vi "BigArraySandbox.vi"() -> ()   [LabVIEW 2016]
panel:
  in  "other Y axis":enum16{"A", "B", "C", "D"}(ring)=enum."D"
  in  "Z Ring":u16(ring) items=["I", "Vsd", "V4T", "dI/dV 2T", "dV/dI 2T", "dV/dI 4T", "dI/dV 4T", "DSA_Vsg1", "B", "B"]
  in  "Scan names 4":string[](array[string])
  in  "Z":T1(ring)
  in  "Y Ring":u16(ring) items=["I", "Vsd", "V4T", "dI/dV 2T", "dV/dI 2T", "dV/dI 4T", "dI/dV 4T", "DSA_Vsg1", "B", "B"]
  in  "Scan names 3":string[](array[string])
  in  "Y":T1(ring)
  in  "X Ring":u16(ring) items=["I", "Vsd", "V4T", "dI/dV 2T", "dV/dI 2T", "dV/dI 4T", "dI/dV 4T", "DSA_Vsg1", "B", "B"]
  in  "Scan names 2":string[](array[string])
  out "error out":errorcluster
  in  "error in (no error)":errorcluster
  in  "X":T1(ring)
  out "Intensity Info OUT":cluster{dbl[], dbl[]}[](array[cluster])
  in  "Big Ol Array IN":T2(array[cluster])
  in  "Slowest Index (Page)":i32
  in  "Slow Index (Row)":dbl
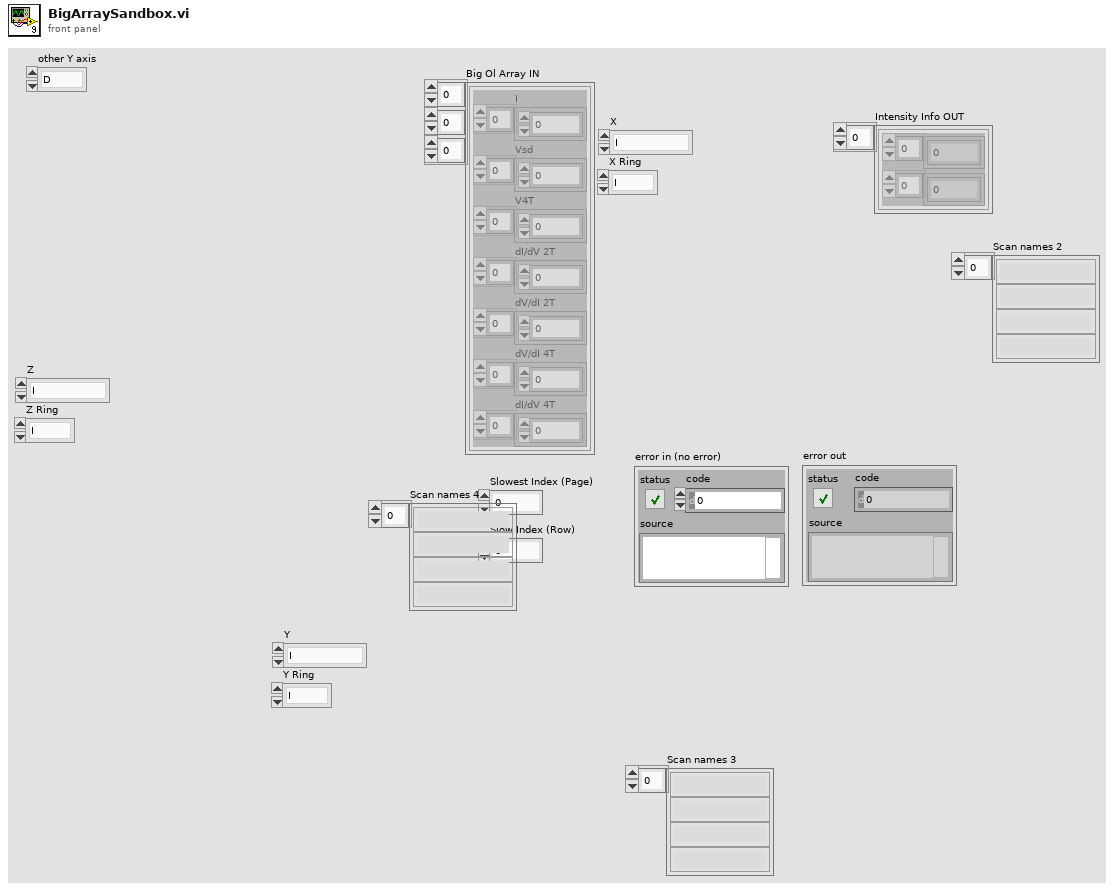
[diagram p1: front panel]
types:
  T1 = enum16{"I", "Vsd", "V4T", "dI/dV 2T", "dV/dI 2T", "dV/dI 4T", "dI/dV 4T"}
  T2 = cluster{"I":dbl[], "Vsd":dbl[], "V4T":dbl[], "dI/dV 2T":dbl[], "dV/dI 2T":dbl[], "dV/dI 4T":dbl[], "dI/dV 4T":dbl[]}[][][]
  T3 = cluster{"I":dbl[], "Vsd":dbl[], "V4T":dbl[], "dI/dV 2T":dbl[], "dV/dI 2T":dbl[], "dV/dI 4T":dbl[], "dI/dV 4T":dbl[]}[]
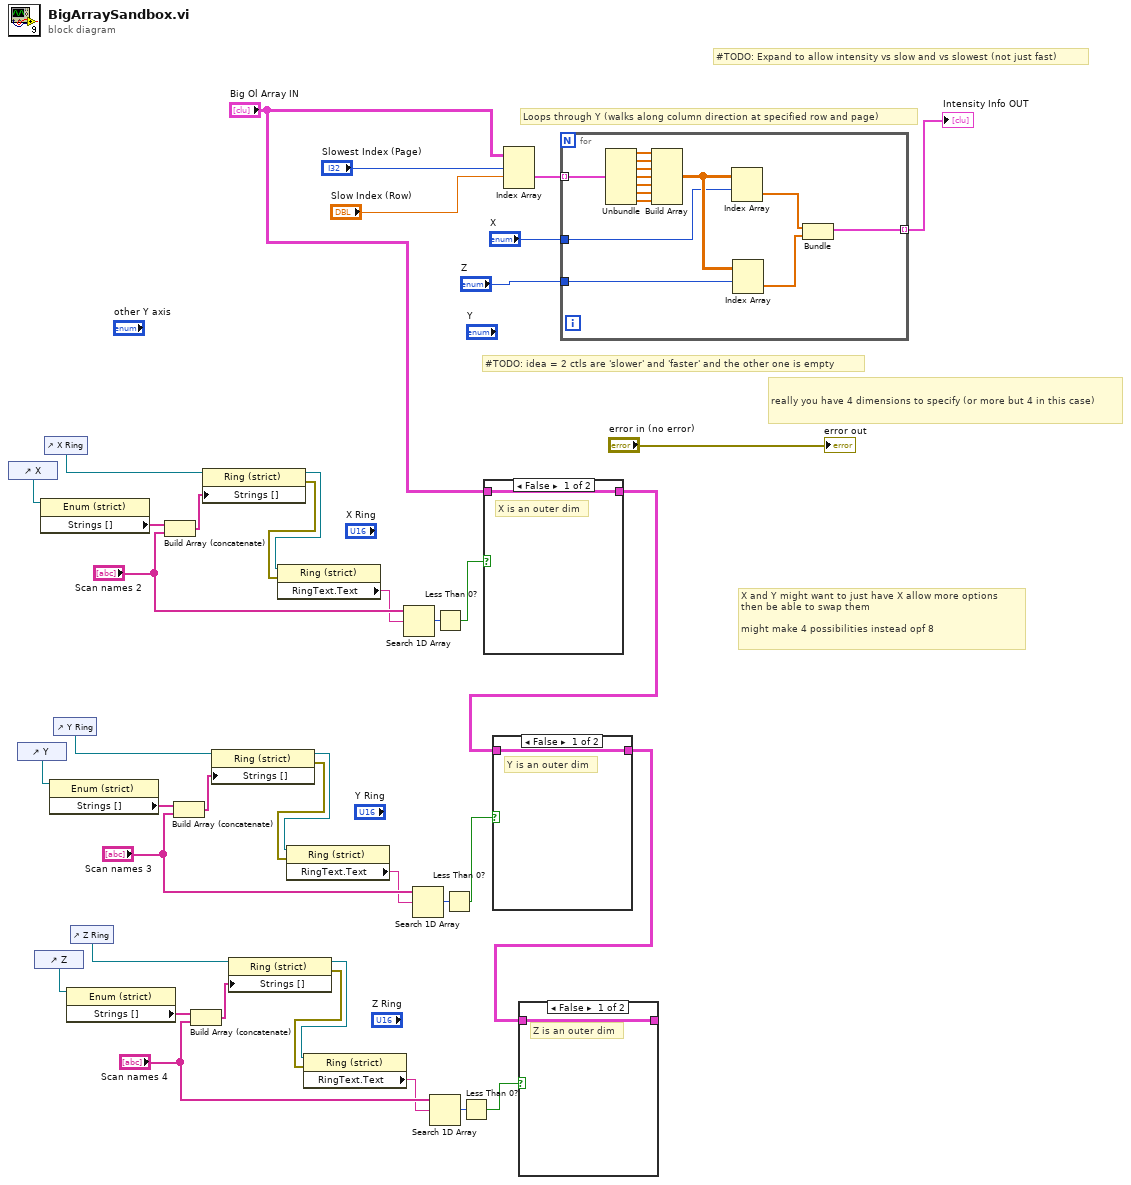
[diagram p0: block diagram]
diagram:
  # "X and Y might want to just have X allow more options\nthen be able to swap them \n\nmight make 4 possibilities instead opf 8"
  # "really you have 4 dimensions to specify (or more but 4 in this case)"
  # "Loops through Y (walks along column direction at specified row and page)"
  # "#TODO: idea = 2 ctls are 'slower' and 'faster' and the other one is empty"
  # "#TODO: Expand to allow intensity vs slow and vs slowest (not just fast)"
  n1 = control-ref of="X"() -> (w24:refnum<vi>)
  n2 = control-ref of="Y"() -> (w15:refnum<vi>)
  n3 = control-ref of="Z"() -> (w6:refnum<vi>)
  n4 = property on="Property Node" class="Enum (strict)"(reference=w24) -> ("Strings []"=w31:string[])  [unwired: 1 in, 2 out]
  n5 = control-ref of="X Ring"() -> (w26:refnum<vi>)
  n6 = property on="Property Node" class="Enum (strict)"(reference=w15) -> ("Strings []"=w21:string[])  [unwired: 1 in, 2 out]
  n7 = control-ref of="Y Ring"() -> (w17:refnum<vi>)
  n8 = property on="Property Node" class="Enum (strict)"(reference=w6) -> ("Strings []"=w12:string[])  [unwired: 1 in, 2 out]
  n9 = control-ref of="Z Ring"() -> (w8:refnum<vi>)
  n10 = Build Array (concatenate)(w31, "Scan names 2") -> (w34:string[])
  n11 = Build Array (concatenate)(w21, "Scan names 3") -> (w23:string[])
  n12 = Build Array (concatenate)(w12, "Scan names 4") -> (w14:string[])
  n13 = property on="Property Node" class="Ring (strict)"(reference=w26, "Strings []"=w34) -> (reference out=w25:refnum<vi>, error out=w33:errorcluster)  [unwired: 1 in]
  n14 = property on="Property Node" class="Ring (strict)"(reference=w17, "Strings []"=w23) -> (reference out=w16:refnum<vi>, error out=w22:errorcluster)  [unwired: 1 in]
  n15 = property on="Property Node" class="Ring (strict)"(reference=w8, "Strings []"=w14) -> (reference out=w7:refnum<vi>, error out=w13:errorcluster)  [unwired: 1 in]
  n16 = property on="Property Node" class="Ring (strict)"(reference=w25, error in=w33) -> ("RingText.Text"=w29:string)  [unwired: 2 out]
  n17 = property on="Property Node" class="Ring (strict)"(reference=w16, error in=w22) -> ("RingText.Text"=w19:string)  [unwired: 2 out]
  n18 = property on="Property Node" class="Ring (strict)"(reference=w7, error in=w13) -> ("RingText.Text"=w10:string)  [unwired: 2 out]
  n19 = Search 1D Array(1D array="Scan names 2", element=w29) -> (index of element=w28:i32)  [unwired: 1 in]
  n20 = Search 1D Array(1D array="Scan names 3", element=w19) -> (index of element=w18:i32)  [unwired: 1 in]
  n21 = Search 1D Array(1D array="Scan names 4", element=w10) -> (index of element=w9:i32)  [unwired: 1 in]
  n22 = Less Than 0?(x=w28) -> (x < 0?=w27:bool)
  n23 = Less Than 0?(x=w18) -> (x < 0?=w4:bool)
  n24 = Less Than 0?(x=w9) -> (x < 0?=w3:bool)
  n25 = case shown="False" w27 {
    tunnel: "Big Ol Array IN" -> [w41 w42]
    tunnel: [w41 w42] -> w2
    frame False {
      # "X is an outer dim"
    }
    frame True {
      # "X is an inner dim"
    }
  }
  n26 = case shown="False" w4 {
    tunnel: w2 -> [w43 w44]
    tunnel: [w43 w44] -> w1
    frame False {
      # "Y is an outer dim"
    }
    frame True {
      # "Y is an inner dim"
    }
  }
  n27 = Index Array(array="Big Ol Array IN", index (dim 0)="Slowest Index (Page)", index (dim 1)="Slow Index (Row)") -> (element=w38:T3)  [unwired: 1 in]
  n28 = case shown="False" w3 {
    tunnel: w1 -> [w45 w46]
    tunnel: [w45 w46] -> _
    frame False {
      # "Z is an outer dim"
    }
    frame True {
      # "Z is an inner dim"
    }
  }
  n29 = for {
    tunnel: w38 -> [w53] mode=indexing
    tunnel: [w49] -> w39 mode=indexing
    tunnel: "X" -> [w48]
    tunnel: "Z" -> [w47]
    n30 = Unbundle(w53) -> ("I"=w60:dbl[], "Vsd"=w59:dbl[], "V4T"=w58:dbl[], "dI/dV 2T"=w57:dbl[], "dV/dI 2T"=w56:dbl[], "dV/dI 4T"=w55:dbl[], "dI/dV 4T"=w54:dbl[])
    n31 = Build Array(w60, w59, w58, w57, w56, w55, w54) -> (w52:dbl[][])
    n32 = Index Array(array=w52, index (row)=w48) -> (element=w50:dbl[])  [unwired: 1 in]
    n33 = Index Array(array=w52, index (row)=w47) -> (element=w51:dbl[])  [unwired: 1 in]
    n34 = Bundle(w50, w51) -> (w49:cluster{dbl[], dbl[]})  [unwired: 1 in]
  }
  "Intensity Info OUT" <- w39
  "error out" <- "error in (no error)"
